vi "ReadM2MaxCurrent.vi"(0 "VISA Refnum in":refnum<visa-resource-name>, 2 "Address":u8, 3 "error in (no error)":errorcluster) -> (1 "MinCurrent":i32, 4 "MaxCurrent":i32, 5 "VISA Refnum out":refnum<visa-resource-name>, 6 "Valid":bool, 8 "error out":errorcluster)   [LabVIEW 2015, in "Ion Motion Roboclaw.lvlib"]
uses:
  <instrlib>/Ion Motion Roboclaw/Ion Motion Roboclaw.lvlib
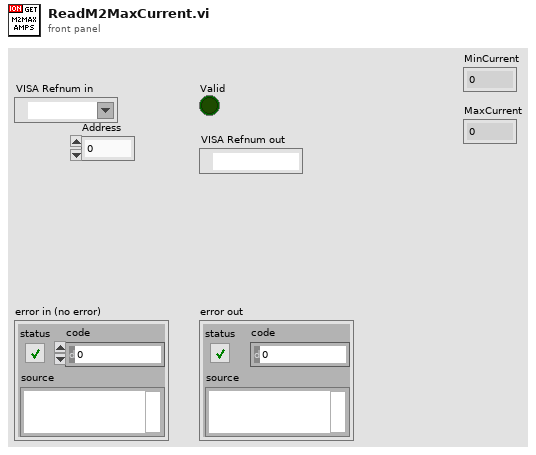
[diagram p1: front panel]
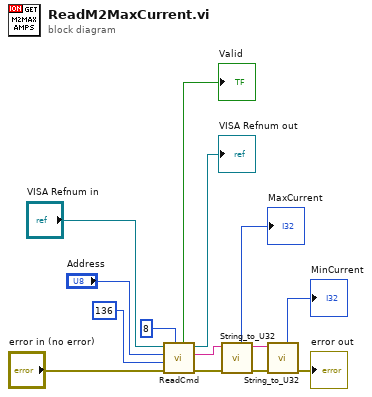
[diagram p0: block diagram]
diagram:
  n1 = call <instrlib>:"ReadCmd.vi"("Read Count"=8 ("cnt"), "error in (no error)"="error in (no error)", "Cmd"=u8 136, "Address"="Address", "VISA Refnum in"="VISA Refnum in") -> ("error out"=w5:errorcluster, "Output"=w6:string, "VISA Refnum out"=→"VISA Refnum out":refnum<visa-resource-name>, "Valid"=→"Valid":bool)  [unwired: 3 in]
  n2 = call <instrlib>:"String_to_U32.vi"("error in (no error)"=w5, "String"=w6) -> ("error out"=w13:errorcluster, "rest of the binary string"=w14:string, "number"=→"MaxCurrent":u32)  [unwired: 5 in]
  n3 = call <instrlib>:"String_to_U32.vi"("error in (no error)"=w13, "String"=w14) -> ("error out"=→"error out":errorcluster, "number"=→"MinCurrent":u32)  [unwired: 5 in, 1 out]
